vi "Teleop.vi"(10 "Match Info":T3={"Autonomous Elapsed Seconds"=0.0, "TeleOp Elapsed Seconds"=0.0, "Disabled Elapsed Seconds"=0.0, "Visited Autonomous"=FALSE, "Visited TeleOp"=FALSE, "Visited Disabled"=FALSE, "Autonomous Settings"={"Autonomous Style"=enum."Independent", "VI Refnum"=refnum}}, 11 "Call Context":T4) -> ()   [LabVIEW 2020]
doc: "This VI is called for each enabled TeleOp packet received from the DS. It is typically used to read from joysticks and other inputs and update I/O or setpoints for timed control loops. It should complete and return within 20 milliseconds or risk missing DS packets."
uses:
  <vilib>/Rock Robotics/WPI/DriverStation/WPI_DriverStationDerivedRobotMode.ctl
  <vilib>/Rock Robotics/WPI/DriverStation/WPI_DriverStationMatch Info.ctl
  <vilib>/Rock Robotics/WPI/Utilities/WPI_GetSetVariantRefNum.vi
  <vilib>/Rock Robotics/Network Tables/NT Write Boolean Array.vi
  <vilib>/Rock Robotics/Network Tables/NT Write Numeric Array.vi
  vi's/Joystick Organization/Joystick Global 6740.vi
  vi's/Global Variables.vi
  <vilib>/Rock Robotics/WPI/ThirdParty/Phoenix-LabVIEW/Motor Controller/Controls/CTRE_Phoenix_MotorControl_ControlMode.ctl
panel:
  in  "set distance":dbl
  in  "output range":cluster{"output high":dbl, "output low":dbl}={"output high"=0.7, "output low"=-0.7} {"output low" format="%.2f"; "output high" format="%.2f"}
  in  "Mode":T1(ring)
  in  "distance PID gains":T2={"proportional gain (Kc)"=0.01, "integral time (Ti, min)"=0.0, "derivative time (Td, min)"=5e-05} {"derivative time (Td, min)" format="%#_6f"}
  in  "angle PID gains":T2={"proportional gain (Kc)"=1.0, "integral time (Ti, min)"=0.0, "derivative time (Td, min)"=0.001}
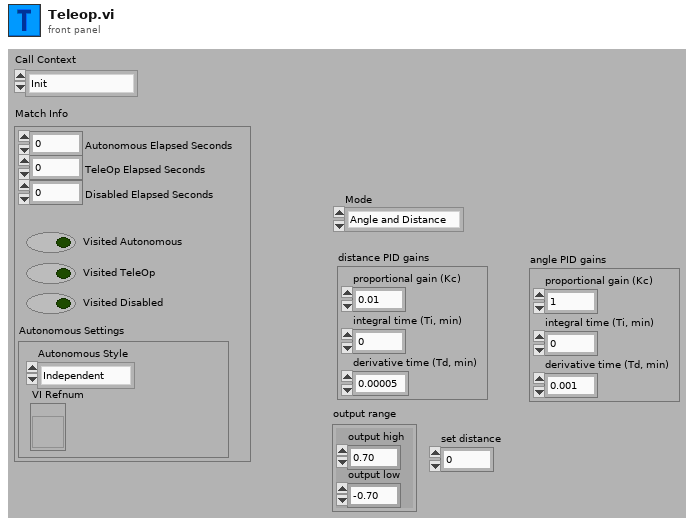
[diagram p1: front panel]
types:
  T1 = enum16{"Angle and Distance", "Distance", "Angle"}
  T2 = cluster{"proportional gain (Kc)":dbl, "integral time (Ti, min)":dbl, "derivative time (Td, min)":dbl}
  T3 = typedef "WPI_DriverStationMatch Info.ctl" = cluster{"Autonomous Elapsed Seconds":dbl, "TeleOp Elapsed Seconds":dbl, "Disabled Elapsed Seconds":dbl, "Visited Autonomous":bool, "Visited TeleOp":bool, "Visited Disabled":bool, "Autonomous Settings":cluster{"Autonomous Style":enum16{"Iterative", "Independent"}, "VI Refnum":refnum<vi>}}
  T4 = typedef "WPI_DriverStationDerivedRobotMode.ctl" = enum16{"Init", "Execute", "Stop"}
  T5 = typedef "CTRE_Phoenix_MotorControl_ControlMode.ctl" = u16
  T6 = typedef "WPI_JoystickDevRef.ctl" = cluster{"Device":T7}
  T7 = typedef "WPI_JoystickDeviceEnum.ctl" = enum16{"USB 0", "USB 1", "USB 2", "USB 3", "USB 4", "USB 5"}
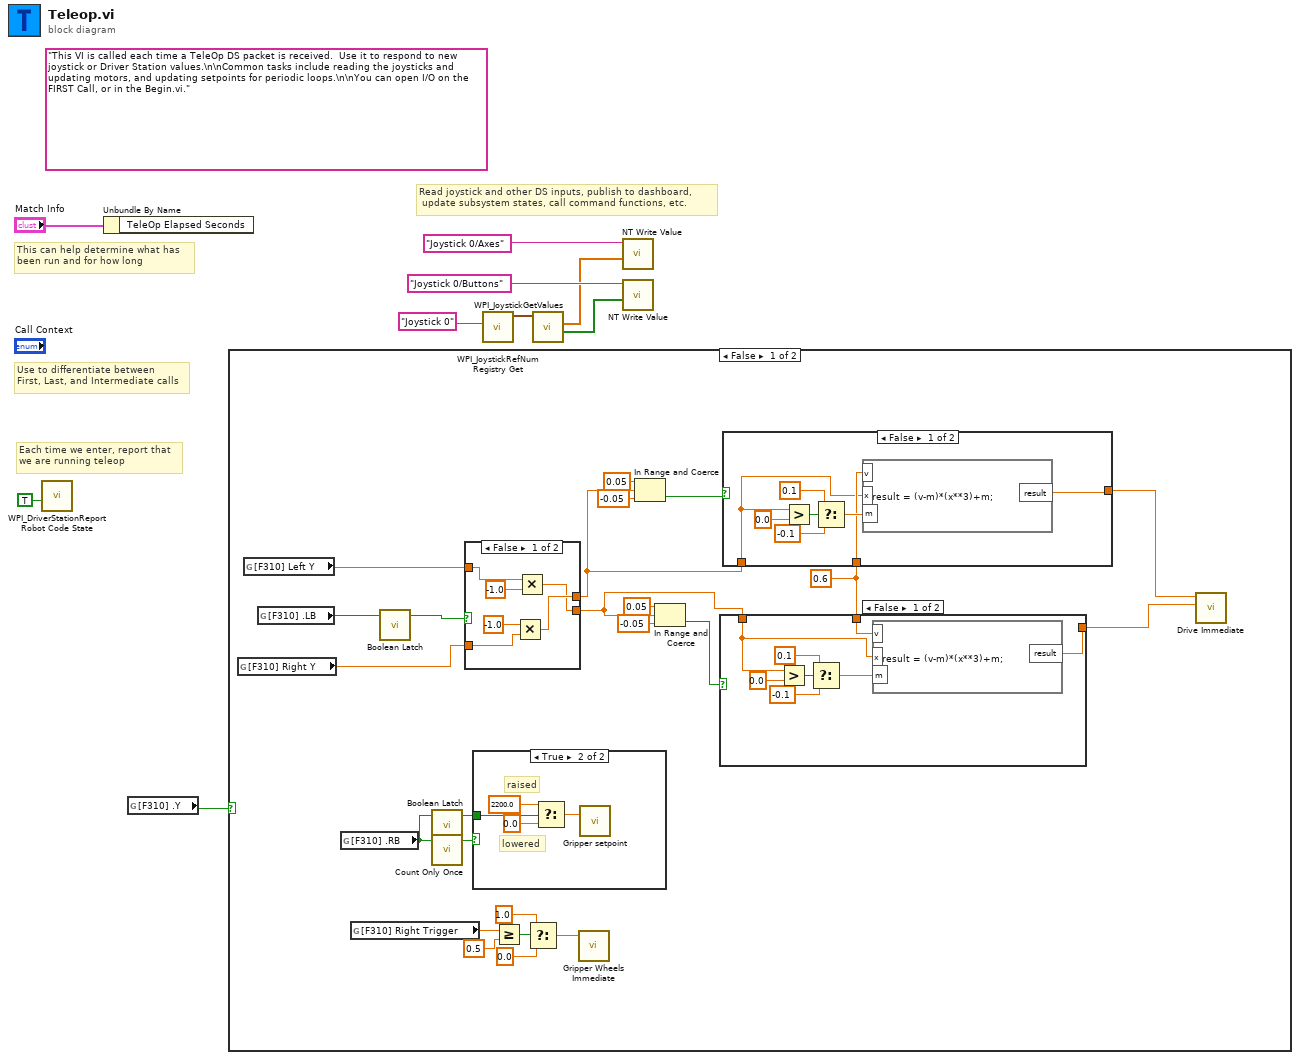
[diagram p0: block diagram]
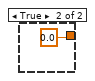
[diagram p2: hidden frame]
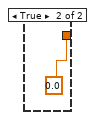
[diagram p3: hidden frame]
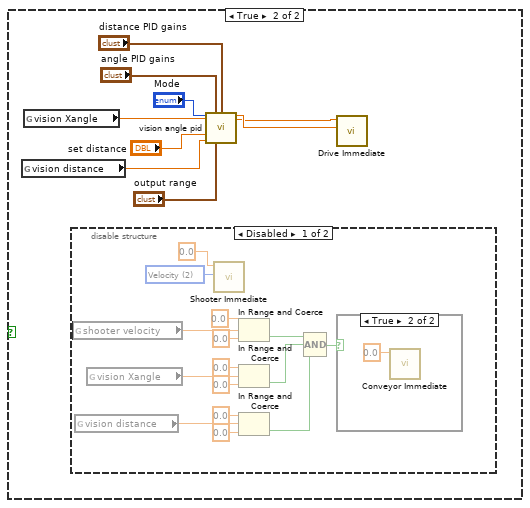
[diagram p6: hidden frame]
diagram:
  (unwired) "This VI is called each time a TeleOp DS packet is received.  Use it to respond to new joystick or Driver Station values.\n\nCommon tasks include reading the joysticks and updating motors, and updating setpoints for periodic loops.\n\nYou can open I/O on the FIRST Call, or in the Begin.vi."
  # "Read joystick and other DS inputs, publish to dashboard,\n update subsystem states, call command functions, etc."
  # "Each time we enter, report that\nwe are running teleop"
  # "Use to differentiate between\nFirst, Last, and Intermediate calls"
  # "This can help determine what has\nbeen run and for how long"
  n1 = call <vilib>:"WPI_DriverStationReport Robot Code State.vi"("TeleOp"=TRUE ("Autonomous")) -> ()  [unwired: 10 in, 1 out]
  n2 = Unbundle By Name("Match Info") -> ()  [unwired: 1 out]
  n3 = global read "Joystick Global 6740.vi" "[F310] .Y"() -> (w1:bool)
  n4 = case shown="False" w1 {
    frame False {
      w16 = 0.6
      n5 = global read "Joystick Global 6740.vi" "[F310] Right Y"() -> (w13:dbl)
      n6 = global read "Joystick Global 6740.vi" "[F310] Left Y"() -> (w15:dbl)
      n7 = global read "Joystick Global 6740.vi" "[F310] .LB"() -> (w29:bool)
      n8 = global read "Joystick Global 6740.vi" "[F310] .RB"() -> (w31:bool)
      n9 = global read "Joystick Global 6740.vi" "[F310] Right Trigger"() -> (w28:dbl)
      n10 = call "Boolean Latch.vi"("Input"=w29) -> ("Output"=w33:bool)  [unwired: 26 in]
      n11 = call "Boolean Latch.vi"("Input"=w31) -> ("Output"=w30:bool)  [unwired: 26 in]
      n12 = call "Count Only Once.vi"("InValue"=w31) -> ("Result"=w32:bool)  [unwired: 26 in]
      n13 = case shown="False" w33 {
        tunnel: w15 -> [w57 w63]
        tunnel: [w58 w62] -> w11
        tunnel: [w59 w63] -> w10
        tunnel: w13 -> [w56 w62]
        frame False {
          n14 = Multiply(x=-1.0, y=w56) -> (x*y=w59:dbl)
          n15 = Multiply(x=w57, y=-1.0) -> (x*y=w58:dbl)
        }
        frame True {
        }
      }
      n16 = case shown="True" w32 {
        tunnel: w30 -> [_ w55]
        frame False {
        }
        frame True {
          # "lowered"
          # "raised"
          n17 = Select(t=2200.0, s=w55, f=0.0) -> (s? t:f=w52:dbl)
          n18 = call "Gripper setpoint.vi"("Setpoint"=w52) -> ()  [unwired: 10 in, 1 out]
        }
      }
      n19 = Greater Or Equal?(x=w28, y=0.5) -> (x >= y?=w25:bool)
      n20 = Select(t=1.0, s=w25, f=0.0) -> (s? t:f=w26:dbl)
      n21 = call "Gripper Wheels Immediate.vi"("Setpoint"=w26) -> ()  [unwired: 10 in, 1 out]
      n22 = In Range and Coerce(upper limit=0.05, x=w10, lower limit=-0.05) -> (In Range?=w14:bool)  [unwired: 1 out]
      n23 = In Range and Coerce(upper limit=0.05, x=w11, lower limit=-0.05) -> (In Range?=w12:bool)  [unwired: 1 out]
      n24 = case shown="False" w12 {
        tunnel: [w36 0.0 ("result")] -> w22
        tunnel: w16 -> [w35 _]
        tunnel: w11 -> [w34 _]
        frame False {
          n25 = Greater?(x=w34, y=0.0) -> (0:w40:bool)
          n26 = Select(t=0.1, s=w40, f=-0.1) -> (s? t:f=w37:dbl)
          n27 = formula code="result = (v-m)*(x**3)+m;"("v"=w35, "x"=w34, "m"=w37) -> ("result"=w36:dbl)
        }
        frame True {
        }
      }
      n28 = case shown="False" w14 {
        tunnel: [w45 0.0 ("result")] -> w21
        tunnel: w16 -> [w44 _]
        tunnel: w10 -> [w43 _]
        frame False {
          n29 = Greater?(x=w43, y=0.0) -> (0:w49:bool)
          n30 = Select(t=0.1, s=w49, f=-0.1) -> (s? t:f=w46:dbl)
          n31 = formula code="result = (v-m)*(x**3)+m;"("v"=w44, "x"=w43, "m"=w46) -> ("result"=w45:dbl)
        }
        frame True {
        }
      }
      n32 = call "Drive Immediate.vi"("Right Setpoint"=w22, "Left Setpoint"=w21) -> ()  [unwired: 9 in, 1 out]
    }
    frame True {
      n33 = global read "Global Variables.vi" "vision distance"() -> (w66:dbl)
      n34 = global read "Global Variables.vi" "vision Xangle"() -> (w68:dbl)
      n35 = disable-structure shown="Disabled" {
        frame Disabled {
          w74 = T5 2 items=["PercentOutput"=0, "Position"=1, "Velocity"=2, "Current"=3, "Follower"=5, "MotionProfile"=6, "MotionMagic"=7, "MotionProfileArc"=10, "Disabled"=15] ("Control Mode")
          n36 = global read "Global Variables.vi" "shooter velocity"() -> (w87:dbl)
          n37 = global read "Global Variables.vi" "vision distance"() -> (w85:dbl)
          n38 = global read "Global Variables.vi" "vision Xangle"() -> (w86:dbl)
          n39 = call "Shooter Immediate.vi"("Control Mode"=w74, "Setpoint"=0.0) -> ()  [unwired: 9 in, 1 out]
          n40 = In Range and Coerce(upper limit=0.0, x=w87, lower limit=0.0) -> (In Range?=w78:bool)  [unwired: 1 out]
          n41 = In Range and Coerce(upper limit=0.0, x=w86, lower limit=0.0) -> (In Range?=w77:bool)  [unwired: 1 out]
          n42 = In Range and Coerce(upper limit=0.0, x=w85, lower limit=0.0) -> (In Range?=w76:bool)  [unwired: 1 out]
          n43 = Compound Arithmetic op=AND(w78, w77, w76) -> (w75:bool)
          n44 = case shown="True" w75 {
            frame False {
            }
            frame True {
              n45 = call "Conveyor Immediate.vi"("Setpoint"=0.0) -> ()  [unwired: 10 in, 1 out]
            }
          }
        }
        frame Enabled {
        }
      }
      n46 = call "vision angle pid.vi"("Mode"="Mode", "angle PID gains"="angle PID gains", "distance PID gains"="distance PID gains", "current angle"=w68, "set distance"="set distance", "current distance"=w66, "output range"="output range") -> ("left velocity"=w65:dbl, "right velocity"=w64:dbl)  [unwired: 7 in]
      n47 = call "Drive Immediate.vi"("Right Setpoint"=w65, "Left Setpoint"=w64) -> ()  [unwired: 9 in, 1 out]
    }
  }
  n48 = call <vilib>:"WPI_JoystickRefNum Registry Get.vi"("refnum name"="Joystick 0") -> ("JoystickDevRef"=w6:T6)  [unwired: 1 in, 9 out]
  n49 = call <vilib>:"WPI_JoystickGetValues.vi"("JoystickDevRef"=w6) -> ("Buttons"=w4:bool[], "Axes"=w3:dbl[])  [unwired: 6 in, 3 out]
  n50 = call-poly <vilib>:"NT Write Value.vi"("Numeric Array"=w3, "Name"="Joystick 0/Axes") -> ()  [unwired: 9 in, 1 out]
  n51 = call-poly <vilib>:"NT Write Value.vi"("Boolean Array"=w4, "Name"="Joystick 0/Buttons") -> ()  [unwired: 9 in, 1 out]
